vi "USB2XXXSPIW25Q32.vi"() -> ()   [LabVIEW 2010]
panel:
  in  "pConfig":T1
  out "Read Data(Hex)":string
  in  "Read Data Count":i32=8
  in  "Start Addr(Hex)":u32 format="%x"
  in  "Write Data(Hex)":string="11 22 33 44 55 66 77 88"
  in  "Channel Index":i32(ring) items=["SPI1_CS0", "SPI2_CS0"]
  in  "Device Index":i32(ring) items=["0", "1", "2", "3", "4", "5"]
  out "Flag(T:Write;F:Read)":bool=TRUE
  in  "stop":bool
  in  "Read":bool
  in  "Write":bool
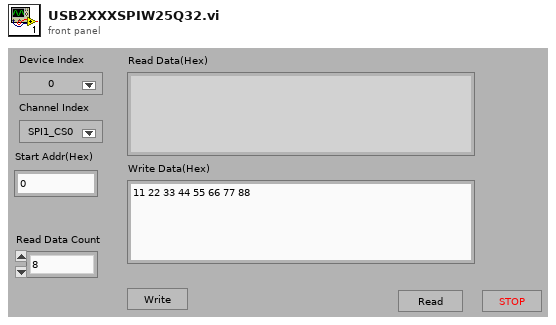
[diagram p1: front panel]
types:
  T1 = cluster{"Mode":i8, "Master":i8, "CPOL":i8, "CPHA":i8, "LSBFirst":i8, "SelPolarity":i8, "@dummy control@":i8, "@dummy control@":i8, "ClockSpeedHz":u32}
  T2 = enum16{"Init", "Write", "Read", "Idel", "Close", "Erase"}
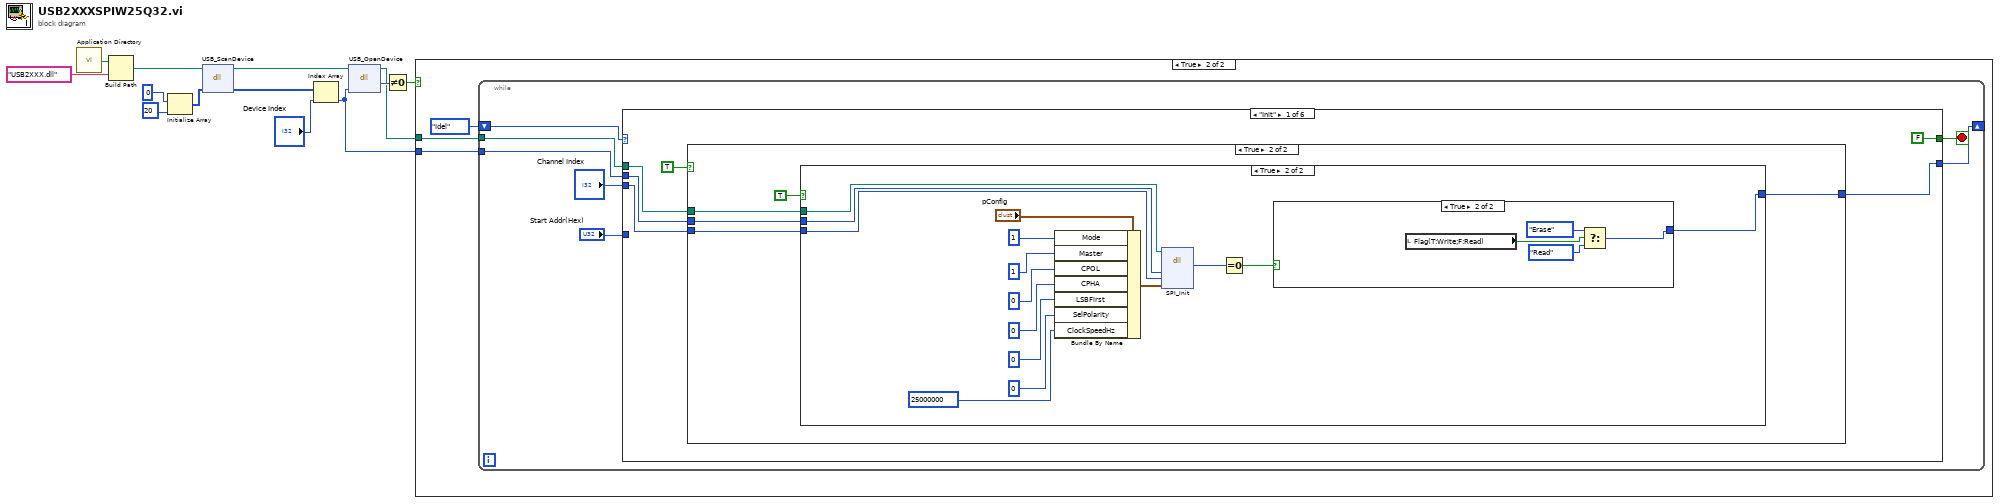
[diagram p0: block diagram]
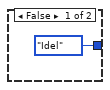
[diagram p3: hidden frame]
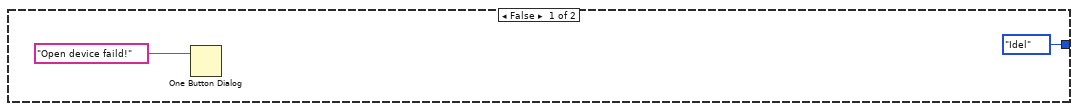
[diagram p4: hidden frame]
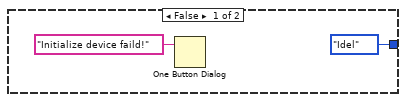
[diagram p5: hidden frame]
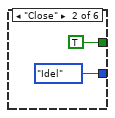
[diagram p6: hidden frame]
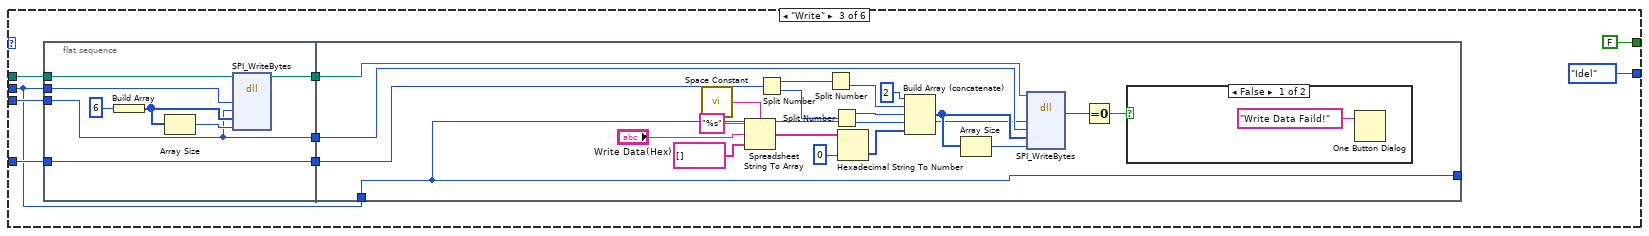
[diagram p7: hidden frame]
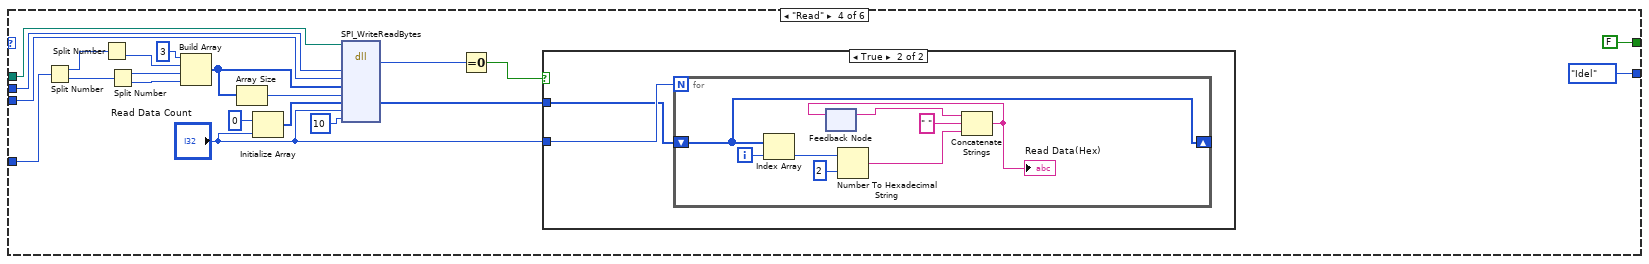
[diagram p9: hidden frame]
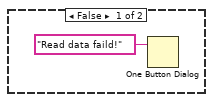
[diagram p10: hidden frame]
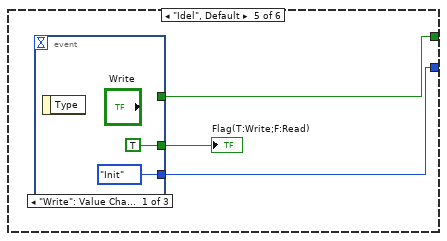
[diagram p11: hidden frame]
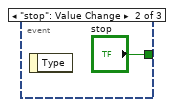
[diagram p12: hidden frame]
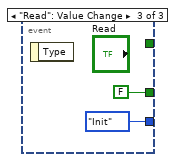
[diagram p13: hidden frame]
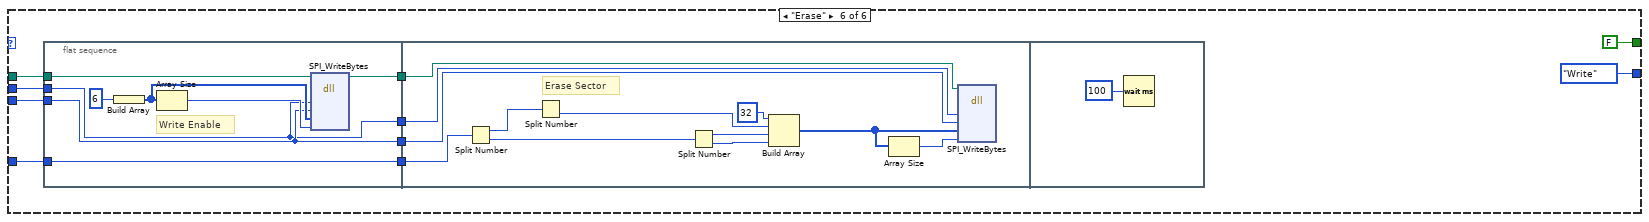
[diagram p14: hidden frame]
diagram:
  n1 = call <vilib>:"Application Directory.vi"() -> ("Application Directory"=w12:path)
  n2 = Build Path(base path=w12, name or relative path="USB2XXX.dll") -> (appended path=w6:path)
  n3 = Initialize Array(0, 20 ("dimension size")) -> (w7:i32[])
  n4 = dll-call lib="E:/Projects/USB2XXX_Example/examples/Labview/USB2SPI/USB2XXX.*" fn="USB_ScanDevice"(path in=w6, "pDevNum"=w7) -> (path out=w5:path, "pDevNum"=w9:i32[])  [unwired: 3 in, 1 out]
  n5 = Index Array(array=w9, index="Device Index") -> (element=w1:i32)
  n6 = dll-call lib="E:/Projects/USB2XXX_Example/examples/Labview/USB2SPI/USB2XXX.*" fn="USB_OpenDevice"(path in=w5, "DevIndex"=w1) -> (path out=w2:path, "return type"=w4:u8)  [unwired: 3 in, 1 out]
  n7 = Not Equal To 0?(x=w4) -> (x != 0?=w3:bool)
  n8 = case shown="True" w3 {
    tunnel: w2 -> [_ w15]
    tunnel: w1 -> [_ w14]
    frame False {
    }
    frame True {
      n9 = while {
        shift-right: [w23] -> _
        shift-left: T2."Idel" ("Enum") -> [w17]
        tunnel: w15 -> [w19]
        tunnel: w14 -> [w18]
        stop <- w20 stop-if-true
        n10 = case shown="\"Init\"" w17 {
          tunnel: [w29 T2."Idel" ("Enum") T2."Idel" ("Enum") T2."Idel" ("Enum") w132 T2."Write" ("Enum")] -> w23
          tunnel: w18 -> [w26 _ w63 w109 _ w148]
          tunnel: "Channel Index" -> [w28 _ w68 w108 _ w147]
          tunnel: "Start Addr(Hex)" -> [_ _ w67 w111 _ w144]
          tunnel: [FALSE TRUE FALSE FALSE w133 FALSE] -> w20
          tunnel: w19 -> [w25 _ w62 w100 _ w140]
          frame "Init" {
            n11 = case shown="True" TRUE {
              tunnel: w26 -> [_ w33]
              tunnel: w28 -> [_ w35]
              tunnel: [T2."Idel" ("Enum") w34] -> w29
              tunnel: w25 -> [_ w32]
              frame False {
              }
              frame True {
                n12 = case shown="True" TRUE {
                  tunnel: w35 -> [_ w50]
                  tunnel: w33 -> [_ w49]
                  tunnel: [T2."Idel" ("Enum") w51] -> w34
                  tunnel: w32 -> [_ w38]
                  frame False {
                    n13 = One Button Dialog(message="Open device faild!") -> ()  [unwired: 1 in, 1 out]
                  }
                  frame True {
                    n14 = Bundle By Name(cluster="pConfig", "Mode"=i8 1, "Master"=i8 1, "CPOL"=i8 0, "CPHA"=i8 0, "LSBFirst"=i8 0, "SelPolarity"=i8 0, "ClockSpeedHz"=u32 25000000) -> (w48:T1)
                    n15 = dll-call lib="E:/Projects/USB2XXX_Example/examples/Labview/USB2SPI/USB2XXX.*" fn="SPI_Init"(path in=w38, "DevIndex"=w49, "SPIIndex"=w50, "pConfig"=w48) -> ("return type"=w47:i32)  [unwired: 5 in, 2 out]
                    n16 = Equal To 0?(x=w47) -> (x = 0?=w52:bool)
                    n17 = case shown="True" w52 {
                      tunnel: [T2."Idel" ("Enum") w57] -> w51
                      frame False {
                        n18 = One Button Dialog(message="Initialize device faild!") -> ()  [unwired: 1 in, 1 out]
                      }
                      frame True {
                        n19 = local read "Flag(T:Write;F:Read)"() -> (w58:bool)
                        n20 = Select(t=T2."Erase" ("Enum"), s=w58, f=T2."Read" ("Enum")) -> (s? t:f=w57:T2)
                      }
                    }
                  }
                }
              }
            }
          }
          frame "Close" {
          }
          frame "Write" {
            n21 = flat-sequence {
              tunnel: w63 -> [w72]
              tunnel: w68 -> [w73]
              tunnel: w67 -> [w74]
              tunnel: [w74] -> w66
              tunnel: [w73] -> w65
              tunnel: w62 -> [w71]
              tunnel: [w70] -> w61
              tunnel: w66 -> [w81]
              tunnel: w65 -> [w80]
              tunnel: [w79] -> _
              tunnel: w63 -> [w79]
              tunnel: w61 -> [w78]
              frame #0 {
                n22 = Build Array(u8 6) -> (w76:u8[])
                n23 = Array Size(array=w76) -> (size(s)=w75:i32)
                n24 = dll-call lib="E:/Projects/USB2XXX_Example/examples/Labview/USB2SPI/USB2XXX.*" fn="SPI_WriteBytes"(path in=w71, "DevIndex"=w72, "SPIIndex"=w73, "pWriteData"=w76, "WriteLen"=w75) -> (path out=w70:path)  [unwired: 7 in, 1 out]
              }
              frame #1 {
                n25 = call <vilib>:"Space Constant.vi"() -> ("String"=w86:string)
                n26 = Spreadsheet String To Array(delimiter (Tab)=w86, format string="%s", spreadsheet string="Write Data(Hex)", array type (2D Dbl)=string[] []) -> (array=w83:string[])
                n27 = Split Number(x=w81) -> (hi(x)=w90:u16, lo(x)=w91:u16)
                n28 = Split Number(x=w90) -> (lo(x)=w92:u8)  [unwired: 1 out]
                n29 = Split Number(x=w91) -> (hi(x)=w93:u8, lo(x)=w94:u8)
                n30 = Hexadecimal String To Number(string=w83, default (0uL)=u8 0 ("default (0 U32)")) -> (number=w95:u8[])  [unwired: 1 in, 1 out]
                n31 = Build Array (concatenate)(u8 2, w92, w93, w94, w95) -> (w98:u8[])
                n32 = Array Size(array=w98) -> (size(s)=w96:i32)
                n33 = dll-call lib="E:/Projects/USB2XXX_Example/examples/Labview/USB2SPI/USB2XXX.*" fn="SPI_WriteBytes"(path in=w78, "DevIndex"=w79, "SPIIndex"=w80, "pWriteData"=w98, "WriteLen"=w96) -> ("return type"=w97:i32)  [unwired: 6 in, 2 out]
                n34 = Equal To 0?(x=w97) -> (x = 0?=w88:bool)
                n35 = case shown="False" w88 {
                  frame False {
                    n36 = One Button Dialog(message="Write Data Faild!") -> ()  [unwired: 1 in, 1 out]
                  }
                  frame True {
                  }
                }
              }
            }
          }
          frame "Read" {
            n37 = Split Number(x=w111) -> (hi(x)=w116:u16, lo(x)=w115:u16)
            n38 = Split Number(x=w116) -> (lo(x)=w114:u8)  [unwired: 1 out]
            n39 = Split Number(x=w115) -> (hi(x)=w113:u8, lo(x)=w112:u8)
            n40 = Build Array(u8 3, w114, w113, w112) -> (w107:u8[])
            n41 = Array Size(array=w107) -> (size(s)=w106:i32)
            n42 = Initialize Array(u8 0 ("element"), "Read Data Count") -> (w105:u8[])
            n43 = dll-call lib="E:/Projects/USB2XXX_Example/examples/Labview/USB2SPI/USB2XXX.*" fn="SPI_WriteReadBytes"(path in=w100, "DevIndex"=w109, "SPIIndex"=w108, "pWriteData"=w107, "WriteLen"=w106, "pReadData"=w105, "ReadLen"="Read Data Count", "IntervalTimeUs"=10 ("TimeOutMs")) -> ("return type"=w110:i32, "pReadData"=w102:u8[])  [unwired: 8 in, 2 out]
            n44 = Equal To 0?(x=w110) -> (x = 0?=w119:bool)
            n45 = case shown="True" w119 {
              tunnel: "Read Data Count" -> [_ w123]
              tunnel: w102 -> [_ w122]
              frame False {
                n46 = One Button Dialog(message="Read data faild!") -> ()  [unwired: 1 in, 1 out]
              }
              frame True {
                n47 = for {
                  N: w123 -> [_]
                  shift-right: [w124] -> _
                  shift-left: w122 -> [w124]
                  i -> [w131]
                  n48 = Index Array(array=w124, index=w131) -> (element=w130:u8)
                  n49 = feedback #1() -> (w128:string)  [unwired: 1 in]
                  n50 = Number To Hexadecimal String(1:i16 2 ("width (-)"), 2:w130) -> (0:w126:string)
                  n51 = Concatenate Strings(w128, " " ("string"), w126) -> (w125:string)
                  "Read Data(Hex)" <- w125
                  n52 = feedback-in #1(w125) -> ()
                }
              }
            }
          }
          frame "Idel", Default {
            n53 = event shown="[0] \"Write\": Value Change" {
              selector: _ -> [_ _ _]
              dyn-events: _ -> [_ _ _]
              timeout: _ -> [_ _ _]
              tunnel: [TRUE _ FALSE] -> w134
              tunnel: [_ "stop" _] -> w133
              tunnel: [T2."Init" ("Enum") _ T2."Init" ("Enum")] -> w132
              event "Write": Value Change {
                n54 = event-data() -> ()  [unwired: 1 in, 1 out]
              }
              event "stop": Value Change {
                n55 = event-data() -> ()  [unwired: 1 in, 1 out]
              }
              event "Read": Value Change {
                n56 = event-data() -> ()  [unwired: 1 in, 1 out]
              }
            }
            "Flag(T:Write;F:Read)" <- w134
          }
          frame "Erase" {
            n57 = flat-sequence {
              tunnel: w148 -> [w153]
              tunnel: w147 -> [w154]
              tunnel: [w154] -> w146
              tunnel: [w153] -> w145
              tunnel: w144 -> [w152]
              tunnel: [w152] -> w143
              tunnel: [w151] -> w141
              tunnel: w140 -> [w150]
              tunnel: w146 -> [w166]
              tunnel: w145 -> [w165]
              tunnel: w143 -> [w164]
              tunnel: w141 -> [w158]
              frame #0 {
                # "Write Enable"
                n58 = Build Array(u8 6) -> (w156:u8[])
                n59 = Array Size(array=w156) -> (size(s)=w155:i32)
                n60 = dll-call lib="E:/Projects/USB2XXX_Example/examples/Labview/USB2SPI/USB2XXX.*" fn="SPI_WriteBytes"(path in=w150, "DevIndex"=w153, "SPIIndex"=w154, "pWriteData"=w156, "WriteLen"=w155) -> (path out=w151:path)  [unwired: 7 in, 1 out]
              }
              frame #1 {
                # "Erase Sector"
                n61 = Split Number(x=w164) -> (hi(x)=w163:u16, lo(x)=w162:u16)
                n62 = Split Number(x=w163) -> (lo(x)=w161:u8)  [unwired: 1 out]
                n63 = Split Number(x=w162) -> (hi(x)=w160:u8, lo(x)=w159:u8)
                n64 = Build Array(u8 32, w161, w160, w159) -> (w168:u8[])
                n65 = Array Size(array=w168) -> (size(s)=w167:i32)
                n66 = dll-call lib="E:/Projects/USB2XXX_Example/examples/Labview/USB2SPI/USB2XXX.*" fn="SPI_WriteBytes"(path in=w158, "DevIndex"=w165, "SPIIndex"=w166, "pWriteData"=w168, "WriteLen"=w167) -> ()  [unwired: 7 in, 2 out]
              }
              frame #2 {
                n67 = Wait (ms)(milliseconds to wait=u32 100) -> ()  [unwired: 1 out]
              }
            }
          }
        }
      }
    }
  }
